vi "update available parameters.vi"(10 "inventory":T1, 11 "Available parameters":refnum<vi>) -> ()   [LabVIEW 2016]
panel:
  in  "id":i32
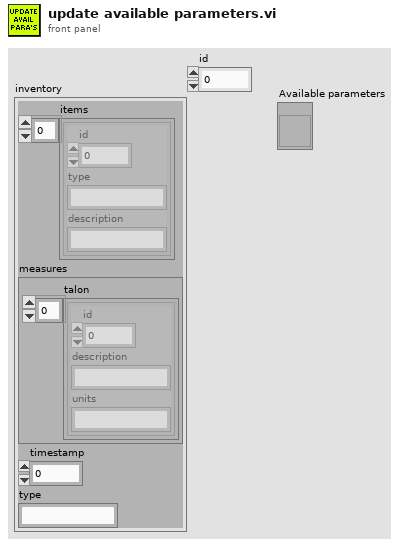
[diagram p1: front panel]
types:
  T1 = cluster{"items":cluster{"id":u8, "type":string, "description":string}[], "measures":cluster{"talon":cluster{"id":u8, "description":string, "units":string}[]}, "timestamp":i32, "type":string}
  T2 = cluster{"id":u8, "description":string, "units":string}[]
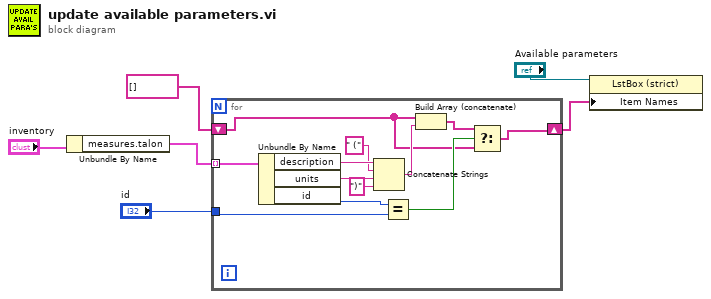
[diagram p0: block diagram]
diagram:
  n1 = Unbundle By Name("inventory") -> ("measures.talon"=w3:T2)
  n2 = for {
    tunnel: "id" -> [w17]
    tunnel: w3 -> [w16] mode=indexing
    shift-right: [w14] -> w1
    shift-left: string[] [] -> [w7]
    n3 = Unbundle By Name(w16) -> ("description"=w13:string, "units"=w12:string, "id"=w18:u8)
    n4 = Concatenate Strings(w13, " (" ("string"), w12, ")" ("string")) -> (w9:string)
    n5 = Equal?(x=w18, y=w17) -> (x = y?=w15:bool)
    n6 = Build Array (concatenate)(w7, w9) -> (w8:string[])
    n7 = Select(t=w8, s=w15, f=w7) -> (s? t:f=w14:string[])
  }
  n8 = property class="LstBox (strict)"(reference="Available parameters", "Item Names"=w1) -> ()  [unwired: 1 in, 2 out]
